vi "HCC Check For Disabled Stations and Get Agilent List.vi"(8 "Error In":errorcluster, 11 "Agilent Channels":string[](array[string])) -> (0 "Error Out":errorcluster, 1 "Voltage Indexes":i32[](array[numeric]), 2 "Agilent Channels DAQ":string="213,214,215,216,217,218,219,220", 3 "Disable Channel = True":bool[](array[boolean])=[TRUE, TRUE, TRUE, TRUE, TRUE, TRUE, TRUE, TRUE, TRUE, TRUE, TRUE, TRUE, FALSE, FALSE, FALSE, FALSE, FALSE, FALSE, FALSE, FALSE, TRUE, TRUE, TRUE, TRUE])   [LabVIEW 2016]
uses:
  <vilib>/Utility/error.llb/whitespace.ctl
  Drivers/Agilent 34972/Agilent 34970.lvlib
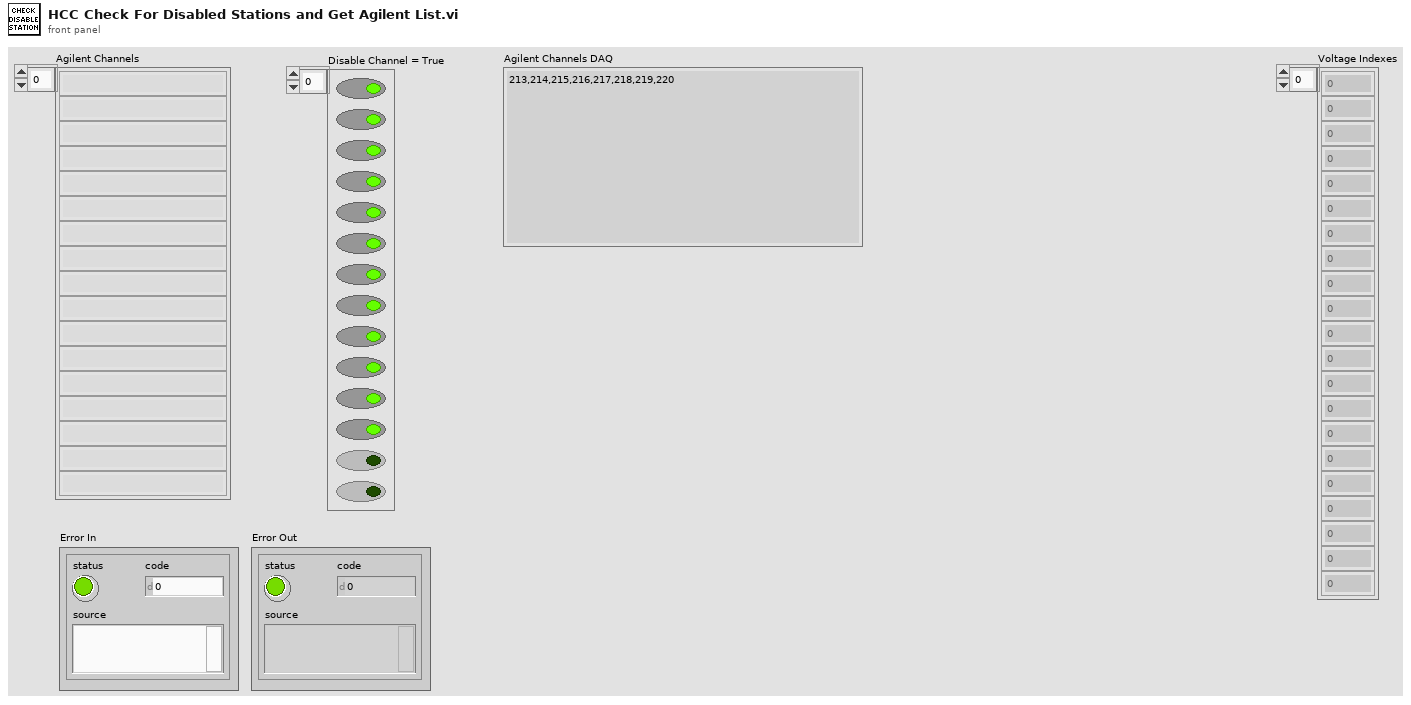
[diagram p1: front panel]
types:
  T1 = typedef "whitespace.ctl" = u16
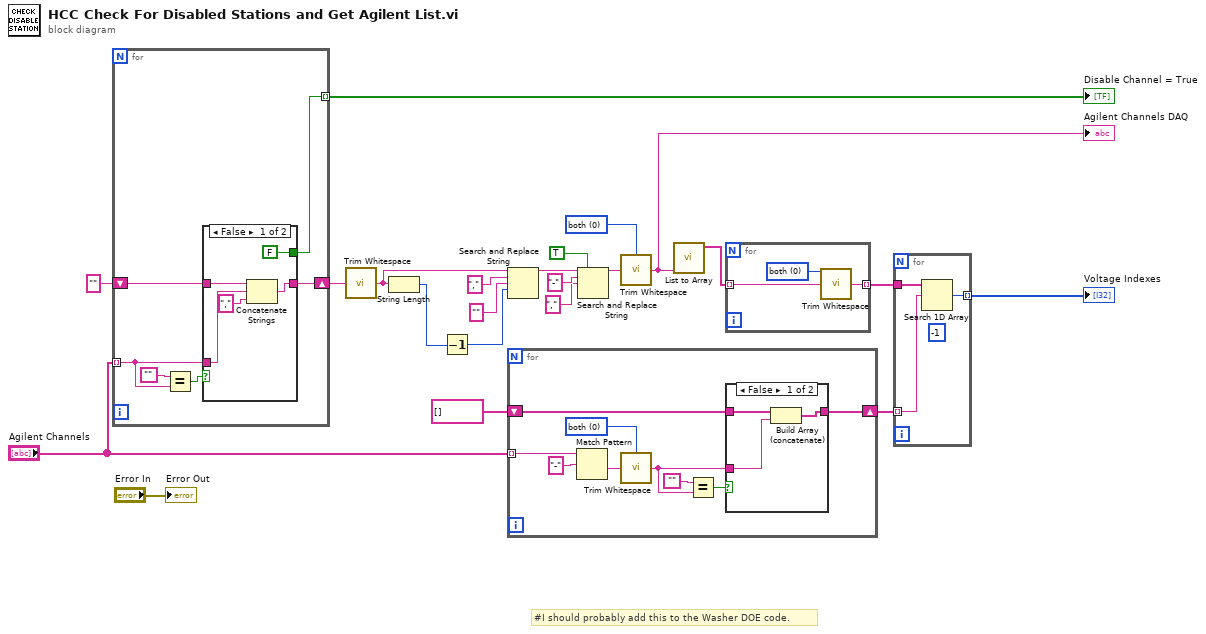
[diagram p0: block diagram]
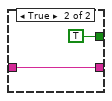
[diagram p3: hidden frame]
diagram:
  w9 = T1 0 items=["both", "start of string", "end of string"] ("location (both)")
  # "#I should probably add this to the Washer DOE code."
  n1 = for {
    tunnel: "Agilent Channels" -> [w25] mode=indexing
    shift-right: [w27] -> w20
    shift-left: "" -> [w28]
    tunnel: [w23] -> w22 mode=indexing
    n2 = Equal?(x="", y=w25) -> (x = y?=w24:bool)
    n3 = case shown="False" w24 {
      tunnel: w28 -> [w33 w35]
      tunnel: w25 -> [w32 _]
      tunnel: [w31 w35] -> w27
      tunnel: [FALSE TRUE] -> w23
      frame False {
        n4 = Concatenate Strings(w33, w32, "," ("string")) -> (w31:string)
      }
      frame True {
      }
    }
  }
  "Disable Channel = True" <- w22
  n5 = call <vilib>:"Trim Whitespace.vi"("string"=w20) -> ("trimmed string"=w15:string)  [unwired: 1 in]
  n6 = String Length(string=w15) -> (length=w19:i32)
  n7 = Decrement(x=w19) -> (x-1=w18:i32)
  n8 = Search and Replace String(input string=w15, search string="," ("string"), replace string="", offset=w18) -> (result string=w8:string)  [unwired: 4 in, 3 out]
  n9 = for {
    tunnel: "Agilent Channels" -> [w44] mode=indexing
    shift-right: [w37] -> w2
    shift-left: string[] [] -> [w38]
    w42 = T1 0 items=["both", "start of string", "end of string"] ("location (both)")
    n10 = Match Pattern(string=w44, regular expression="-") -> (after substring=w41:string)  [unwired: 1 in, 3 out]
    n11 = call <vilib>:"Trim Whitespace.vi"("string"=w41, "location (both)"=w42) -> ("trimmed string"=w36:string)
    n12 = Equal?(x="", y=w36) -> (x = y?=w39:bool)
    n13 = case shown="False" w39 {
      tunnel: w38 -> [w47 w48]
      tunnel: [w46 w48] -> w37
      tunnel: w36 -> [w45 _]
      frame False {
        n14 = Build Array (concatenate)(w47, w45) -> (w46:string[])
      }
      frame True {
      }
    }
  }
  n15 = Search and Replace String(replace all?=TRUE ("replace all? (F)"), input string=w8, search string="-", replace string="," ("string")) -> (result string=w10:string)  [unwired: 4 in, 3 out]
  n16 = call <vilib>:"Trim Whitespace.vi"("string"=w10, "location (both)"=w9) -> ("trimmed string"=w6:string)
  "Agilent Channels DAQ" <- w6
  n17 = call "List to Array.vi"("List (empty)"=w6) -> ("Output String Array"=w5:string[])  [unwired: 9 in, 1 out]
  n18 = for {
    tunnel: w5 -> [w50] mode=indexing
    tunnel: [w49] -> w3 mode=indexing
    w51 = T1 0 items=["both", "start of string", "end of string"] ("location (both)")
    n19 = call <vilib>:"Trim Whitespace.vi"("string"=w50, "location (both)"=w51) -> ("trimmed string"=w49:string)
  }
  n20 = for {
    tunnel: w3 -> [w54]
    tunnel: w2 -> [w53] mode=indexing
    tunnel: [w52] -> w1 mode=indexing
    (unwired) -1 ("y")
    n21 = Search 1D Array(1D array=w54, element=w53) -> (index of element=w52:i32)  [unwired: 1 in]
  }
  "Voltage Indexes" <- w1
  "Error Out" <- "Error In"
